vi "Check Configuration Valid.vi"(8 "error in (no error)":errorcluster, 11 "Session in":refnum<class "Session.lvclass">) -> (0 "error out":errorcluster, 2 "Configuration Valid?":bool, 3 "Session out":refnum<class "Session.lvclass">)   [LabVIEW 2020, in "HTTP Server.lvlib" / "Session.lvclass"]
uses:
  Session.lvclass
  Session.lvclass/Session.ctl
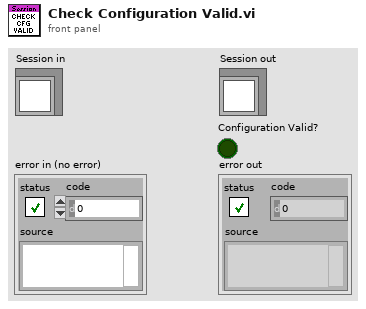
[diagram p1: front panel]
types:
  T1 = enum16{"open", "replace", "create", "open or create", "replace or create", "replace or create with confirmation"}
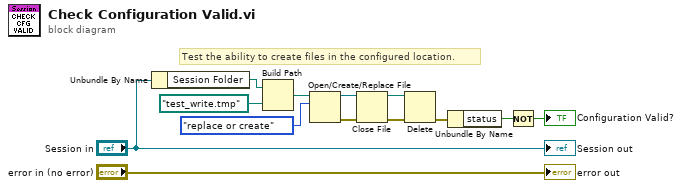
[diagram p0: block diagram]
diagram:
  # "Test the ability to create files in the configured location."
  n1 = Unbundle By Name("Session in") -> ("Session Folder"=w11:path)
  n2 = Build Path(base path=w11, name or relative path=path "test_write.tmp") -> (appended path=w9:path)
  n3 = Open/Create/Replace File(file path (use dialog)=w9, operation (0:open)=T1."replace or create") -> (refnum out=w6:refnum<file>, error out=w7:errorcluster)  [unwired: 4 in, 1 out]
  n4 = Close File(refnum=w6, error in=w7) -> (path=w3:path, error out=w2:errorcluster)
  n5 = Delete(path (use dialog)=w3, error in=w2) -> (error out=w1:errorcluster)  [unwired: 3 in, 2 out]
  n6 = Unbundle By Name(w1) -> ("status"=w5:bool)
  n7 = Not(x=w5) -> (.not. x?=→"Configuration Valid?":bool)
  "error out" <- "error in (no error)"
  "Session out" <- "Session in"
